vi "Two Chart Temple.vi"(8 "error in (no error)":errorcluster caption="错误输入（无错误）") -> (0 "error out":errorcluster caption="错误输出")   [LabVIEW 2015]
doc: "该连续测量范例项目在队列消息处理器模板的基础上实现。\n\n事件处理循环负责按用户界面操作生成对应的消息。\n\n消息处理循环负责对事件处理循环或其他消息生成的消息进行处理。其中还包括用于采集和记录消息处理循环的子VI，以及用于更新图表的循环。"
uses:
  controls/UI Data.ctl
  Measure Type.ctl
  controls/ValueUI Data.ctl
  support/Message Queue/Enqueue Message (Single).vi
  Acquisition/Acquisition.lvlib
  Logging/Logging.lvlib
  support/User Event - Stop/User Event - Stop.lvlib
  support/Message Queue/Message Queue.lvlib
  Action/Action.lvlib
panel:
  out "XY Graph":cluster{"Y":dbl[], "Y":dbl[]}[](graph) caption="XY图"
  out "XY Graph 2":cluster{"Y":dbl[], "Y":dbl[]}[](graph) caption="XY图"
  in  "设置":bool
  in  "清零":bool
  in  "读取":bool
  out "模拟通道5":dbl
  out "模拟通道4":dbl
  out "模拟通道3":dbl
  out "模拟通道2":dbl
  out "模拟通道1":dbl
  out "模拟通道0":dbl
  out "角度":dbl
  in  "计算":bool
  in  "Start":bool caption="开始"
  in  "Stop":bool caption="停止"
  out "Status":string caption="状态"
  in  "Exit":bool caption="退出"
  # "测量项目"
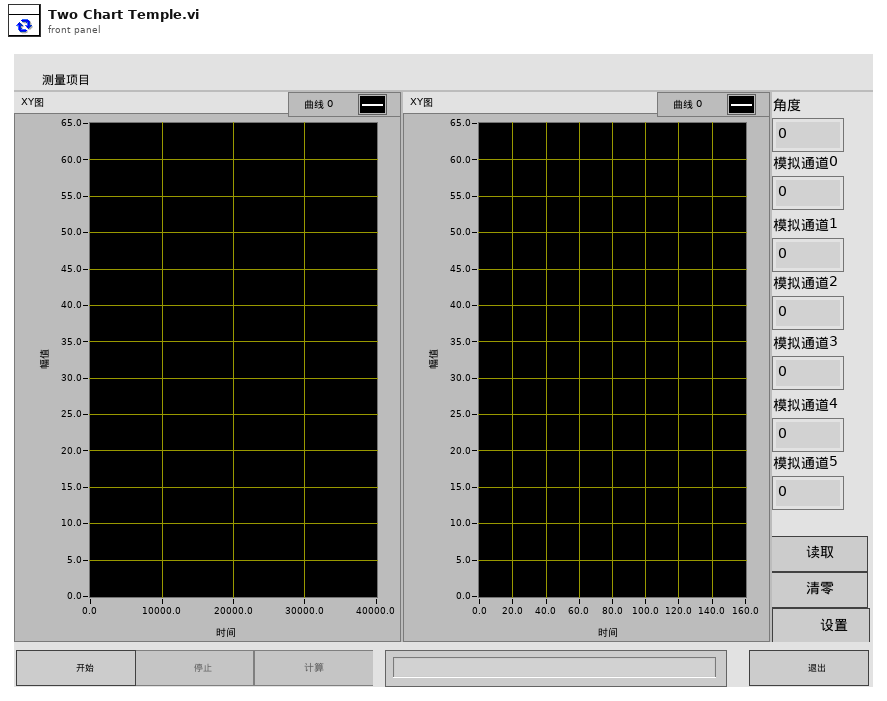
[diagram p1: front panel]
types:
  T1 = typedef "ValueUI Data.ctl" = cluster{"数据1引用":refnum<vi>, "数据2引用":refnum<vi>, "数据3引用":refnum<vi>, "传感器0引用":refnum<vi>, "传感器1引用":refnum<vi>, "传感器2引用":refnum<vi>, "传感器3引用":refnum<vi>, "传感器4引用":refnum<vi>, "传感器5引用":refnum<vi>, "传感器6引用":refnum<vi>}
  T2 = typedef "Measure Type.ctl" = enum16{"啮合", "退回", "功能", "力特性", "内泄漏", "自动调阀测试"}
  T3 = typedef "UI Data.ctl" = cluster{"Start Ref":refnum<vi>, "Stop Ref":refnum<vi>, "calculate Ref":refnum<vi>, "Status Ref":refnum<vi>, "Exit Ref":refnum<vi>, "read Ref":refnum<vi>, "clean Ref":refnum<vi>}
  T4 = typedef "Message Queue.lvlib/All Message Queues.ctl" = cluster{"UI":refnum<queue>, "Acquisition":refnum<queue>, "Logging":refnum<queue>, "plot logic":refnum<queue>, "Action Control":refnum<queue>}
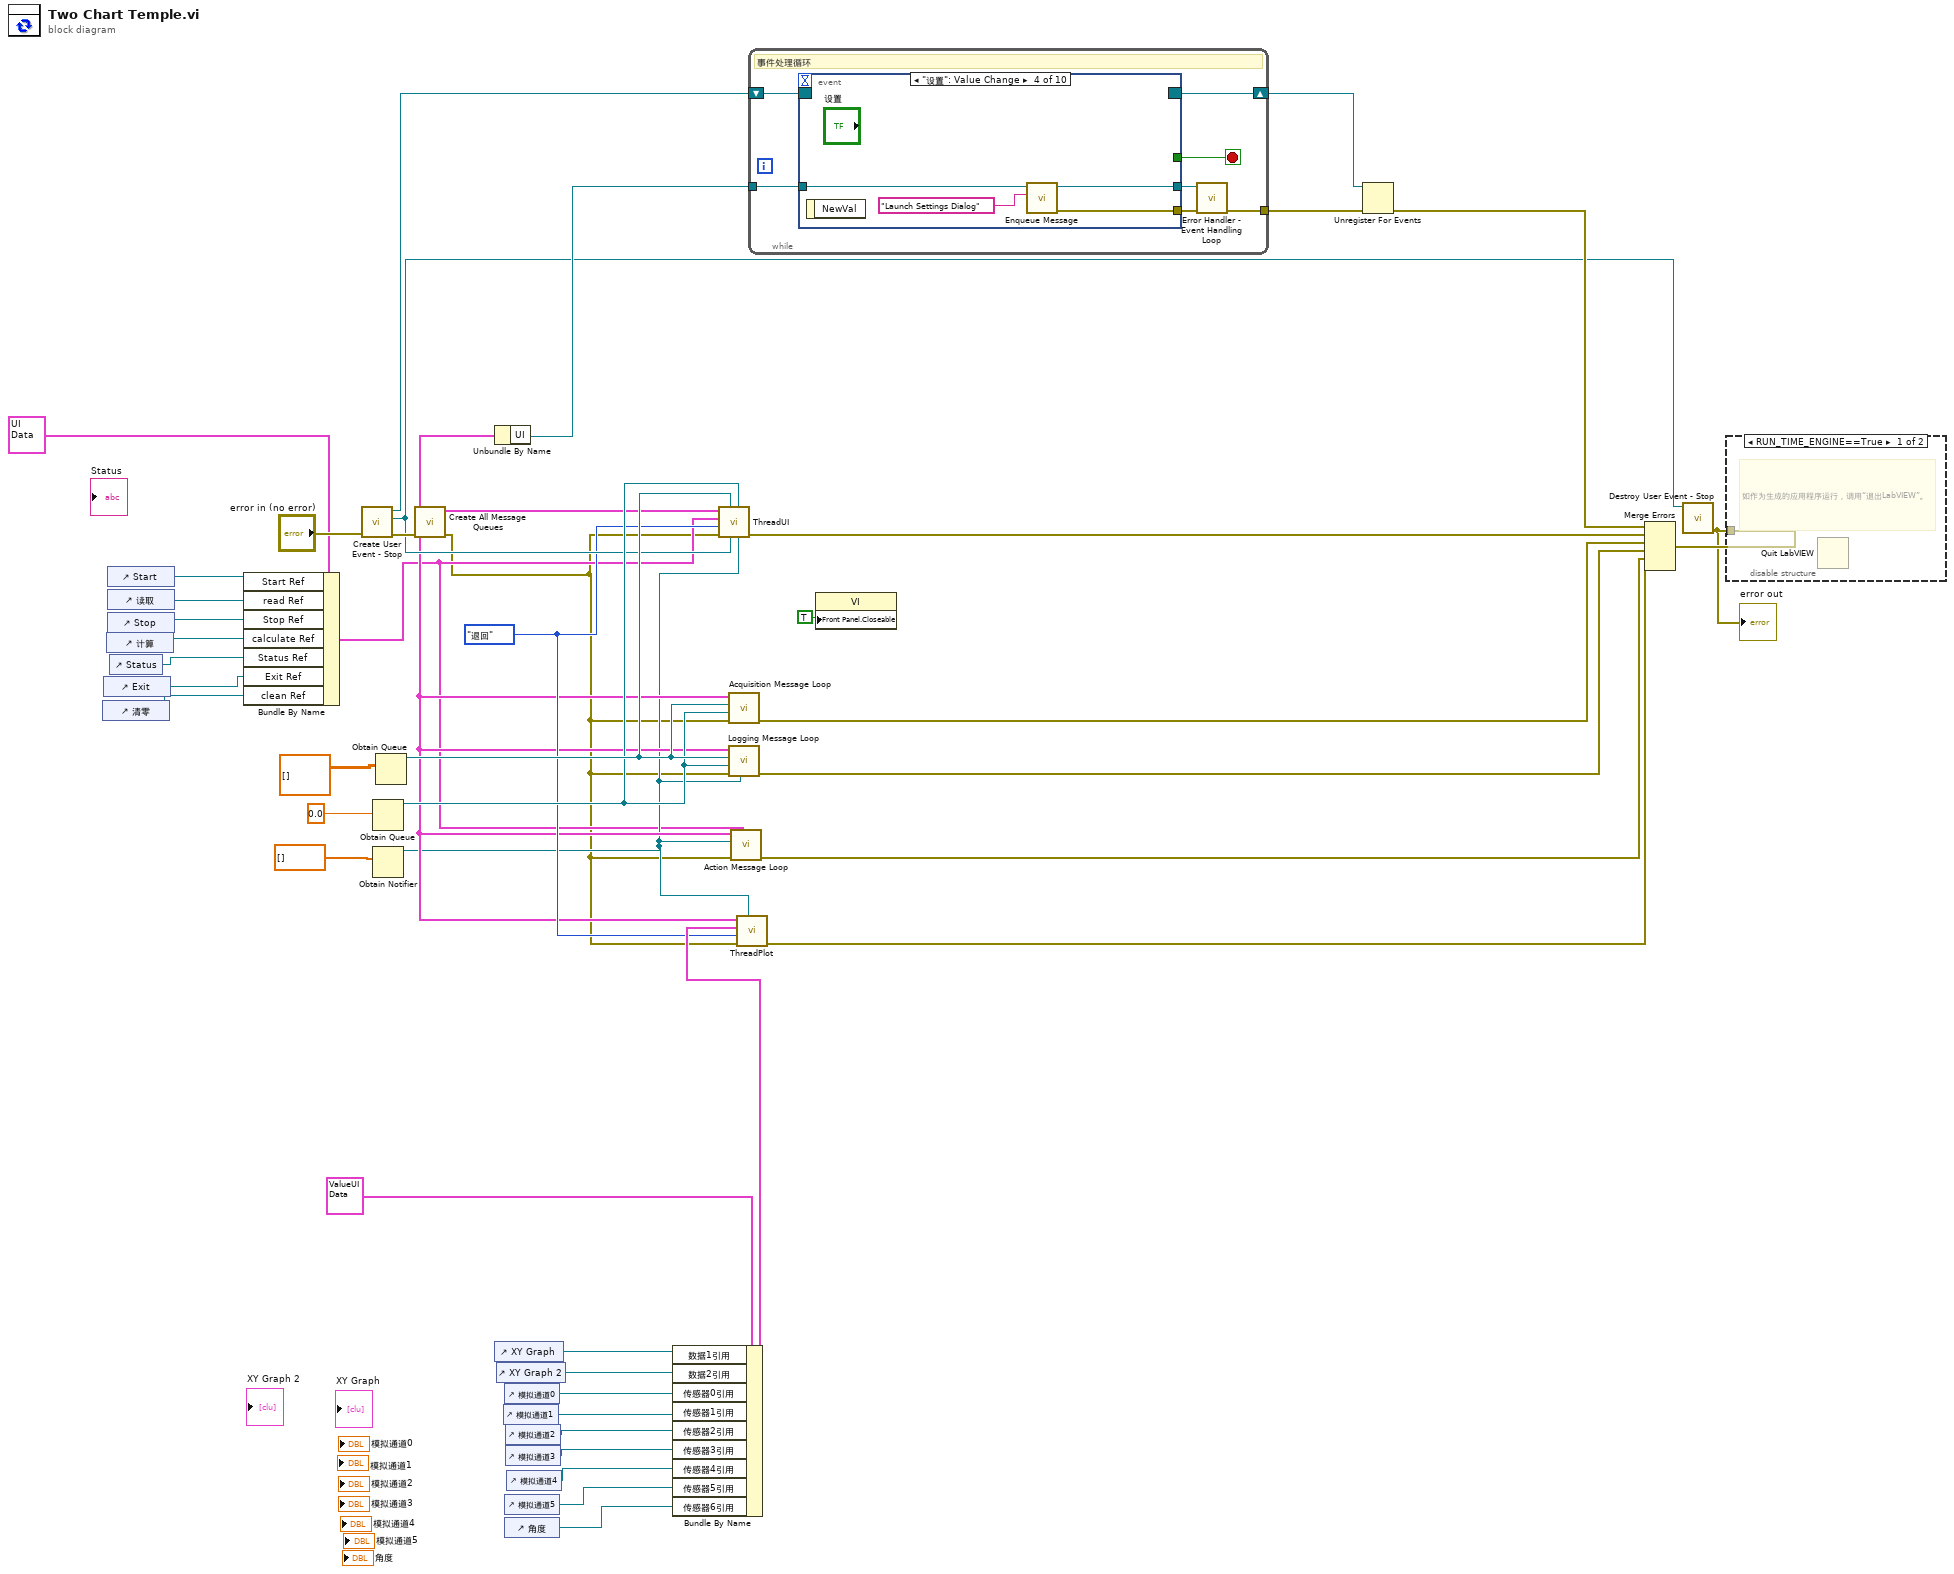
[diagram p0: block diagram]
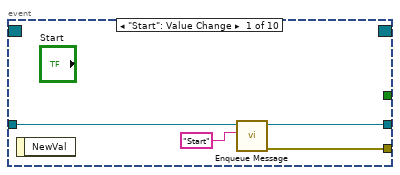
[diagram p3: hidden frame]
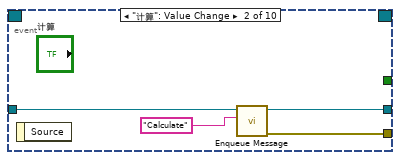
[diagram p4: hidden frame]
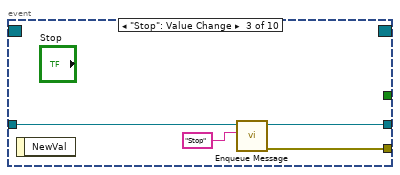
[diagram p5: hidden frame]
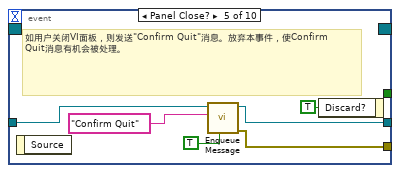
[diagram p6: hidden frame]
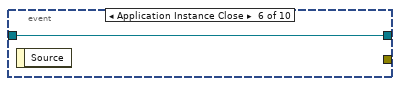
[diagram p7: hidden frame]
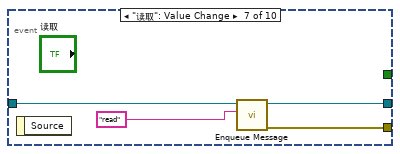
[diagram p8: hidden frame]
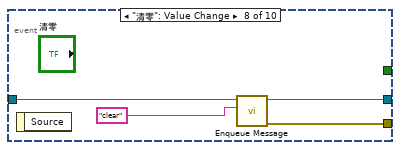
[diagram p9: hidden frame]
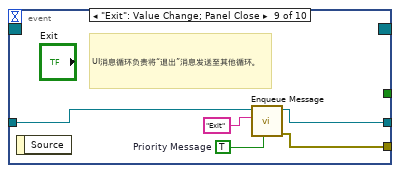
[diagram p10: hidden frame]
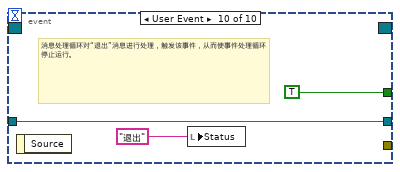
[diagram p11: hidden frame]
diagram:
  w9 = Measure_Type."退回" ("测试类型")
  n1 = control-ref of="清零"() -> (w26:refnum<vi>)
  n2 = control-ref of="Exit"() -> (w29:refnum<vi>)
  n3 = control-ref of="计算"() -> (w25:refnum<vi>)
  n4 = control-ref of="Start"() -> (w31:refnum<vi>)
  n5 = control-ref of="读取"() -> (w27:refnum<vi>)
  n6 = control-ref of="Stop"() -> (w28:refnum<vi>)
  n7 = control-ref of="Status"() -> (w7:refnum<vi>)
  n8 = Bundle By Name(cluster=T3 {"Start Ref"=refnum, "Stop Ref"=refnum, "calculate Ref"=refnum, "Status Ref"=refnum, "Exit Ref"=refnum, "read Ref"=refnum, "clean Ref"=refnum} ("Measurement UI Controls"), "Start Ref"=w31, "read Ref"=w27, "Stop Ref"=w28, "calculate Ref"=w25, "Status Ref"=w7, "Exit Ref"=w29, "clean Ref"=w26) -> (w3:T3)
  n9 = call "Create User Event - Stop.vi"("error in (no error)"="error in (no error)") -> ("error out"=w41:errorcluster, "User Event - Stop"=w21:refnum<user-event>, "Stop Event Registration Refnum"=w43:refnum<event-registration>)  [unwired: 8 in]
  n10 = Obtain Queue(element data type=0.0) -> (queue out=w23:refnum<queue>)  [unwired: 4 in, 2 out]
  n11 = Obtain Notifier(notification data type=dbl[] []) -> (notifier out=w4:refnum<notifier>)  [unwired: 3 in, 2 out]
  n12 = Obtain Queue(element data type=dbl[][] []) -> (queue out=w24:refnum<queue>)  [unwired: 4 in, 2 out]
  n13 = call "Create All Message Queues.vi"("error in (no error)"=w41) -> ("error out"=w2:errorcluster, "Message Queues out"=w5:T4)  [unwired: 9 in]
  n14 = Unbundle By Name(w5) -> ("UI"=w37:refnum<queue>)
  n15 = control-ref of="XY Graph"() -> (w6:refnum<vi>)
  n16 = control-ref of="XY Graph 2"() -> (w18:refnum<vi>)
  n17 = control-ref of="模拟通道1"() -> (w16:refnum<vi>)
  n18 = control-ref of="模拟通道0"() -> (w17:refnum<vi>)
  n19 = control-ref of="模拟通道5"() -> (w12:refnum<vi>)
  n20 = control-ref of="角度"() -> (w11:refnum<vi>)
  n21 = control-ref of="模拟通道2"() -> (w15:refnum<vi>)
  n22 = control-ref of="模拟通道3"() -> (w14:refnum<vi>)
  n23 = control-ref of="模拟通道4"() -> (w13:refnum<vi>)
  n24 = Bundle By Name(cluster=T1 {"数据1引用"=refnum, "数据2引用"=refnum, "数据3引用"=refnum, "传感器0引用"=refnum, "传感器1引用"=refnum, "传感器2引用"=refnum, "传感器3引用"=refnum, "传感器4引用"=refnum, "传感器5引用"=refnum, "传感器6引用"=refnum} ("传感器显示UI控件"), "数据1引用"=w6, "数据2引用"=w18, "传感器0引用"=w17, "传感器1引用"=w16, "传感器2引用"=w15, "传感器3引用"=w14, "传感器4引用"=w13, "传感器5引用"=w12, "传感器6引用"=w11) -> (w10:T1)
  n25 = call "ThreadUI.vi"("数据通知器"=w4, "Angle Data Queue"=w23, "User Event - Stop"=w21, "Analog Data Queue"=w24, "error in (no error)"=w2, "测试类型"=w9, "Measurement UI Controls"=w3, "Message Queues"=w5) -> ("error out"=w20:errorcluster)  [unwired: 3 in]
  n26 = call "Acquisition Message Loop.vi"("error in (no error)"=w2, "Angle Data Queue"=w23, "Analog Data Queue"=w24, "Message Queues"=w5) -> ("error out"=w42:errorcluster)  [unwired: 7 in]
  n27 = call "Logging Message Loop.vi"("数据通知器"=w4, "error in (no error)"=w2, "Angle Data Queue"=w23, "Analog Data Queue"=w24, "Message Queues"=w5) -> ("error out"=w40:errorcluster)  [unwired: 6 in]
  n28 = call "Action Message Loop.vi"("Measurement UI Controls"=w3, "error in (no error)"=w2, "Data Notifier"=w4, "Message Queues"=w5) -> ("error out"=w1:errorcluster)  [unwired: 7 in]
  n29 = call "ThreadPlot.vi"("数据通知器"=w4, "error in (no error)"=w2, "测试类型"=w9, "传感器显示UI控件"=w10, "Message Queues"=w5) -> ("error out"=w8:errorcluster)  [unwired: 6 in]
  n30 = while {
    tunnel: w37 -> [w51]
    tunnel: [w46] -> w45
    shift-right: [w50] -> w38
    shift-left: w43 -> [w52]
    stop <- w49 stop-if-true
    # "事件处理循环"
    n31 = event shown="[3] \"设置\": Value Change" {
      selector: w52 -> [_ _ _ _ _ _ _ _ _ _]
      dyn-events: [_ _ _ _ _ _ _ _ _ _] -> w50
      timeout: _ -> [_ _ _ _ _ _ _ _ _ _]
      tunnel: [_ _ _ _ _ _ _ _ _ TRUE ("Discard?")] -> w49
      tunnel: w51 -> [w54 w59 w63 w67 w74 w75 w77 w81 w85 w89]
      tunnel: [w56 w58 w62 w66 w69 _ w79 w83 w88 _] -> w47
      tunnel: [w53 w57 w61 w65 w70 w75 w76 w80 w84 w89] -> w48
      event "Start": Value Change {
        n32 = event-data() -> ()  [unwired: 1 in, 1 out]
        n33 = call-poly "Enqueue Message.vi"("Message"="Start", "Message Queue"=w54) -> ("error out"=w56:errorcluster, "dup Message Queue"=w53:refnum<queue>)  [unwired: 8 in]
      }
      event "计算": Value Change {
        n34 = event-data() -> ()  [unwired: 1 in, 1 out]
        n35 = call-poly "Enqueue Message.vi"("Message"="Calculate", "Message Queue"=w59) -> ("error out"=w58:errorcluster, "dup Message Queue"=w57:refnum<queue>)  [unwired: 8 in]
      }
      event "Stop": Value Change {
        n36 = event-data() -> ()  [unwired: 1 in, 1 out]
        n37 = call-poly "Enqueue Message.vi"("Message"="Stop", "Message Queue"=w63) -> ("error out"=w62:errorcluster, "dup Message Queue"=w61:refnum<queue>)  [unwired: 8 in]
      }
      event "设置": Value Change {
        n38 = event-data() -> ()  [unwired: 1 in, 1 out]
        n39 = call-poly "Enqueue Message.vi"("Message"="Launch Settings Dialog", "Message Queue"=w67) -> ("error out"=w66:errorcluster, "dup Message Queue"=w65:refnum<queue>)  [unwired: 8 in]
      }
      event Panel Close? {
        # "如用户关闭VI面板，则发送\"Confirm Quit\"消息。放弃本事件，使Confirm Quit消息有机会被处理。"
        n40 = event-data() -> ()  [unwired: 1 in, 1 out]
        n41 = call-poly "Enqueue Message.vi"("Priority Message? (F)"=TRUE, "Message"="Confirm Quit", "Message Queue"=w74) -> ("error out"=w69:errorcluster, "dup Message Queue"=w70:refnum<queue>)  [unwired: 7 in]
        n42 = event-data("Discard?"=TRUE) -> ()  [unwired: 1 in, 1 out]
      }
      event Application Instance Close {
        n43 = event-data() -> ()  [unwired: 1 in, 1 out]
      }
      event "读取": Value Change {
        n44 = event-data() -> ()  [unwired: 1 in, 1 out]
        n45 = call-poly "Enqueue Message.vi"("Message"="read", "Message Queue"=w77) -> ("error out"=w79:errorcluster, "dup Message Queue"=w76:refnum<queue>)  [unwired: 8 in]
      }
      event "清零": Value Change {
        n46 = event-data() -> ()  [unwired: 1 in, 1 out]
        n47 = call-poly "Enqueue Message.vi"("Message"="clear", "Message Queue"=w81) -> ("error out"=w83:errorcluster, "dup Message Queue"=w80:refnum<queue>)  [unwired: 8 in]
      }
      event "Exit": Value Change; Panel Close {
        w86 = TRUE  # Priority Message
        # "UI消息循环负责将“退出”消息发送至其他循环。"
        n48 = event-data() -> ()  [unwired: 1 in, 1 out]
        n49 = call-poly "Enqueue Message.vi"("Priority Message? (F)"=w86, "Message"="Exit", "Message Queue"=w85) -> ("error out"=w88:errorcluster, "dup Message Queue"=w84:refnum<queue>)  [unwired: 7 in]
      }
      event User Event {
        # "消息处理循环对“退出”消息进行处理，触发该事件，从而使事件处理循环停止运行。"
        n50 = event-data() -> ()  [unwired: 1 in, 1 out]
        n51 = local write "Status"("退出" ("Exit String")) -> ()
      }
    }
    n52 = call "Error Handler - Event Handling Loop.vi"("error in (no error)"=w47, "Message Queue"=w48) -> ("dup error in"=w46:errorcluster)  [unwired: 8 in, 1 out]
  }
  n53 = property class="VI"("Front Panel.Closeable"=TRUE ("Front Panel Window:Closeable")) -> ()  [unwired: 2 in, 2 out]
  n54 = Unregister For Events(event registration refnum=w38, error in=w45) -> (error out=w39:errorcluster)
  n55 = Merge Errors(w39, w20, w42, w40, w1, w8) -> (w44:errorcluster)
  n56 = call "Destroy User Event - Stop.vi"("error in (no error)"=w44, "User Event - Stop"=w21) -> ("error out"=w33:errorcluster)  [unwired: 9 in]
  "error out" <- w33
  n57 = disable-structure shown="RUN_TIME_ENGINE==True" {
    disable-tunnel: w33 -> [_ _]
    frame condition #0 {
      # "如作为生成的应用程序运行，调用“退出LabVIEW”。"
      n58 = Quit LabVIEW() -> ()  [unwired: 1 in]
    }
    frame condition #1 (active) {
    }
  }
